vi "Read Roles.vi"(8 "error in (no error)":errorcluster, 11 "TableWithStrikerPlay in":refnum<class "TableWithStrikerPlay.lvclass">) -> (0 "error out":errorcluster, 2 "Roles":T1, 3 "TableWithStrikerPlay out":refnum<class "TableWithStrikerPlay.lvclass">)   [LabVIEW 2021, in "TableWithStrikerPlay.lvclass"]
uses:
  TableWithStrikerPlay.lvclass
  TableFinalizerRole_class/TableFinalizerRole.lvclass
  TablerRole_class/TablerRole.lvclass
  PassObserverRole_class/PassObserverRole.lvclass
  TableWithStrikerPlay.lvclass/TableWithStrikerPlay.ctl
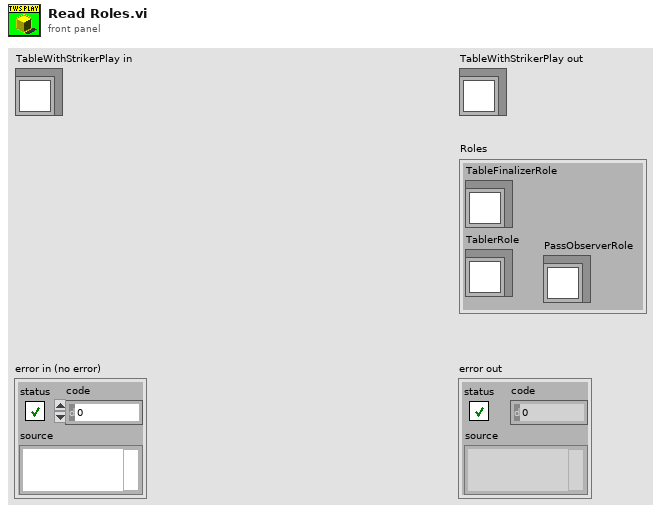
[diagram p1: front panel]
types:
  T1 = cluster{"TableFinalizerRole":refnum<class "TableFinalizerRole.lvclass">, "TablerRole":refnum<class "TablerRole.lvclass">, "PassObserverRole":refnum<class "PassObserverRole.lvclass">}
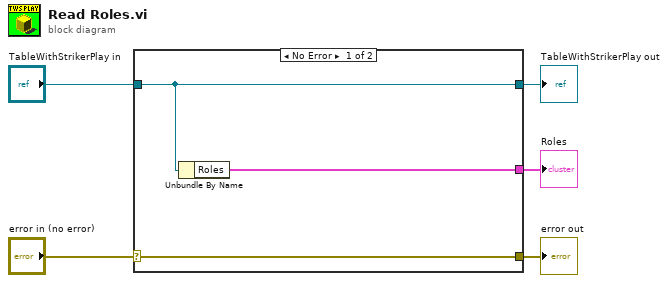
[diagram p0: block diagram]
diagram:
  n1 = case shown="No Error" "error in (no error)" {
    selector: "error in (no error)" -> [w8 w9]
    tunnel: [w8 w9] -> w4
    tunnel: [w7 w10] -> w2
    tunnel: "TableWithStrikerPlay in" -> [w7 w10]
    tunnel: [w6 _] -> w1
    frame No Error {
      n2 = Unbundle By Name(w7) -> ("Roles"=w6:T1)
    }
    frame Error {
    }
  }
  "error out" <- w4
  "TableWithStrikerPlay out" <- w2
  "Roles" <- w1
